vi "GetCCIDInfo.vi"(5 "table name":string="CCID", 6 "Slot":T1, 10 "SerNO":string, 11 "CCID":string) -> (2 "CCID信息":string[](array[string]))   [LabVIEW 2013]
uses:
  SystemCode/SysControl/Slot.ctl
  GlobalValue.vi
panel:
  out "x >= y? 2":bool
  out "子数组":string[](array[string])
  out "x = y?":bool
  out "x >= y?":bool
  out "SerNO OUT":string[](array[string])
  out "CCID 2":string
  out "ID":string
  out "SerNO":string
  out "OUTdata":string[][](array[string])
  out "MainViPath":path
  out "error out":errorcluster caption="错误输出"
  in  "error in (no error)":errorcluster caption="错误输入（无错误）"
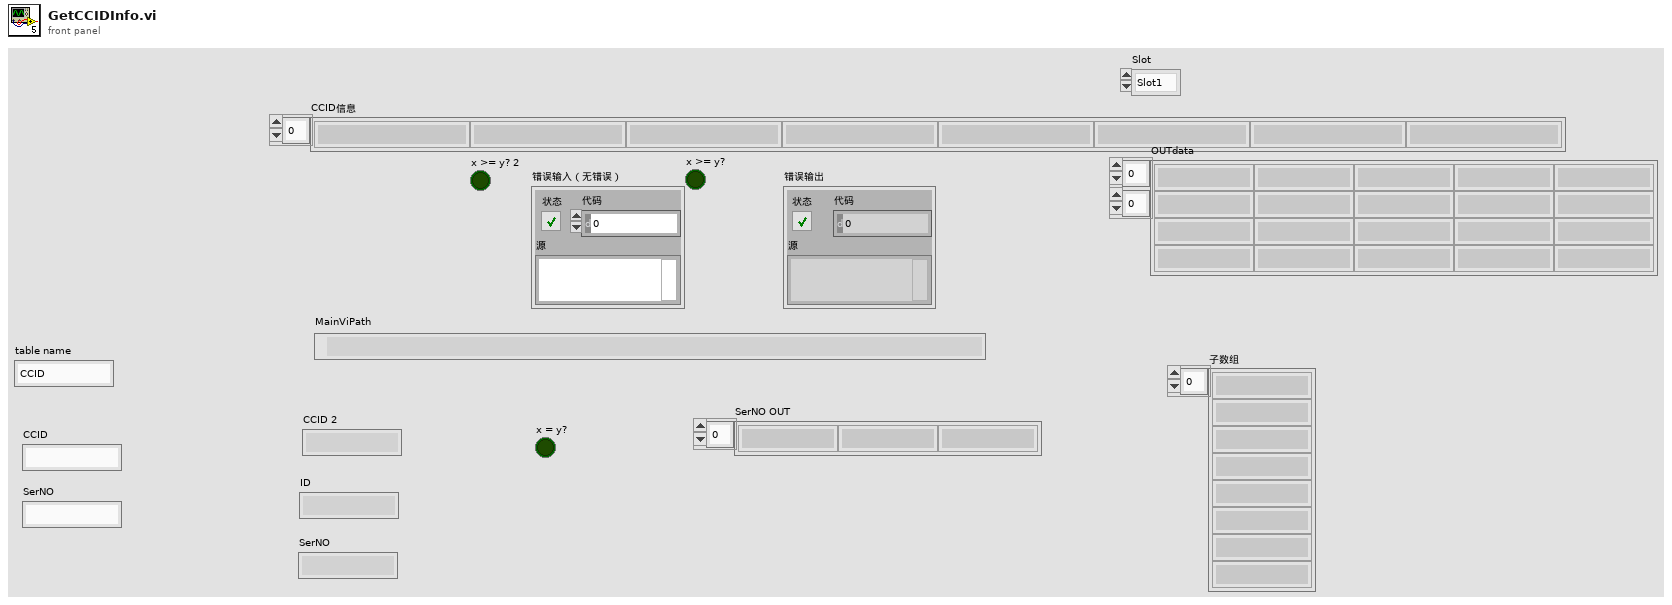
[diagram p1: front panel]
types:
  T1 = typedef "Slot.ctl" = enum16{"Slot1", "Slot2", "Slot3", "Slot4"}
  T2 = enum16{"open", "replace", "create", "open or create", "replace or create", "replace or create with confirmation"}
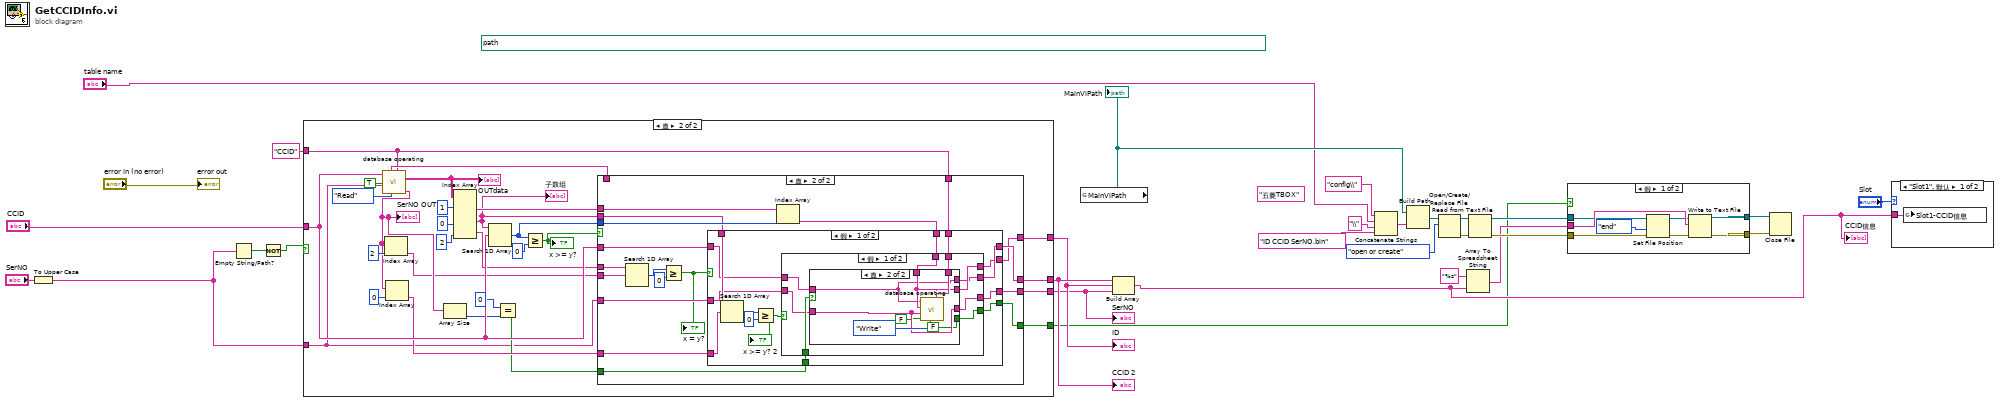
[diagram p0: block diagram]
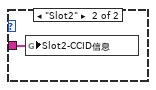
[diagram p3: hidden frame]
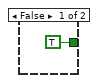
[diagram p4: hidden frame]
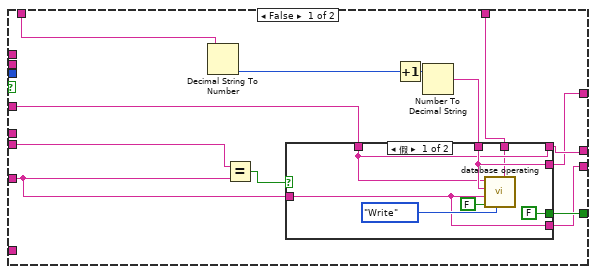
[diagram p5: hidden frame]
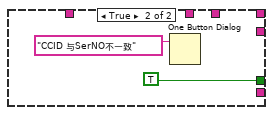
[diagram p6: hidden frame]
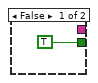
[diagram p7: hidden frame]
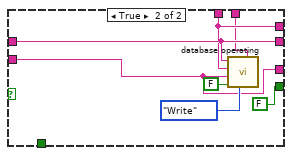
[diagram p8: hidden frame]
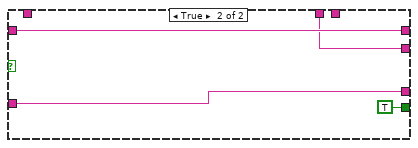
[diagram p9: hidden frame]
diagram:
  (unwired) "五菱TBOX" ("字符串")
  (unwired) path "C:/Documents and Settings/DELL/桌面/homework/五菱T-BOX labview 设计/成品测试/2016-0831 new version/五菱T-BOX TestSystem(增加硬件版本)/五菱T-BOX TestSystem(增加硬件版本)" ("基路径")
  n1 = To Upper Case(1:"SerNO") -> (0:w21:string)
  n2 = Empty String/Path?(string/path=w21) -> (empty?=w23:bool)
  n3 = Not(x=w23) -> (.not. x?=w22:bool)
  n4 = case shown="真" w22 {
    tunnel: "CCID" -> [_ w43]
    tunnel: [_ w57] -> w27
    tunnel: [_ w56] -> w26
    tunnel: [_ w55] -> w25
    tunnel: [TRUE w54] -> w4
    tunnel: w21 -> [_ w32]
    tunnel: "CCID" -> [_ w33]
    frame False {
    }
    frame True {
      n5 = call "database operating.vi"("table name"=w33, "Read or Write"=enum16{"Read", "Write"}."Read", "布尔"=TRUE, "SerNO"=w32, "CCID"=w43) -> ("SerNO OUT"=w38:string[], "OUTdata"=w49:string[][], "OUT MAXID"=w53:string)  [unwired: 4 in]
      "OUTdata" <- w49
      "SerNO OUT" <- w38
      n6 = Index Array(array=w38, index=2 ("索引")) -> (element=w31:string)
      n7 = Index Array(array=w38, index=0 ("索引")) -> (element=w39:string)
      n8 = Array Size(array=w38) -> (size(s)=w37:i32)
      n9 = Index Array(array=w49, index (col) #1=1 ("禁用的索引 (列)"), index (col) #2=0 ("索引 (列)"), index (col) #3=2 ("索引 (列)")) -> (element #1=w48:string[], element #2=w41:string[], element #3=w42:string[])  [unwired: 3 in]
      "子数组" <- w41
      n10 = Search 1D Array(1D array=w41, element=w43) -> (index of element=w50:i32)  [unwired: 1 in]
      n11 = Equal?(x=0, y=w37) -> (x = y?=w35:bool)
      n12 = Greater Or Equal?(x=w50, y=0) -> (x >= y?=w51:bool)
      "x >= y?" <- w51
      n13 = case shown="真" w51 {
        tunnel: w50 -> [_ w92]
        tunnel: w43 -> [w69 w91]
        tunnel: w32 -> [w62 w90]
        tunnel: [w67 w97] -> w57
        tunnel: [w59 w96] -> w56
        tunnel: [w66 w95] -> w55
        tunnel: [w70 w94] -> w54
        tunnel: w53 -> [w65 _]
        tunnel: w48 -> [_ w93]
        tunnel: w42 -> [_ w89]
        tunnel: w31 -> [w63 w84]
        tunnel: w41 -> [_ w85]
        tunnel: w39 -> [_ w83]
        tunnel: w35 -> [_ w82]
        tunnel: w33 -> [w60 w81]
        frame False {
          n14 = Decimal String To Number(string=w65) -> (number=w64:i32)  [unwired: 2 in, 1 out]
          n15 = Equal?(x=w63, y=w62) -> (x = y?=w61:bool)
          n16 = Increment(x=w64) -> (x+1=w71:i32)
          n17 = Number To Decimal String(number=w71) -> (decimal integer string=w68:string)  [unwired: 1 in]
          n18 = case shown="假" w61 {
            tunnel: [FALSE TRUE] -> w70
            tunnel: w69 -> [w75 _]
            tunnel: w68 -> [w77 _]
            tunnel: w62 -> [w74 _]
            tunnel: [w77 _] -> w59
            tunnel: [w75 _] -> w67
            tunnel: [w74 _] -> w66
            tunnel: w60 -> [w72 _]
            frame False {
              n19 = call "database operating.vi"("table name"=w72, "Read or Write"=enum16{"Read", "Write"}."Write", "布尔"=FALSE, "SerNO"=w74, "ID"=w77, "CCID"=w75) -> ()  [unwired: 3 in, 3 out]
            }
            frame True {
              n20 = One Button Dialog(message="CCID 与SerNO不一致" ("消息")) -> ()  [unwired: 1 in, 1 out]
            }
          }
        }
        frame True {
          n21 = Search 1D Array(1D array=w89, element=w84) -> (index of element=w88:i32)  [unwired: 1 in]
          n22 = Greater Or Equal?(x=w88, y=0) -> (x >= y?=w86:bool)
          "x = y?" <- w86
          n23 = Index Array(array=w93, index=w92) -> (element=w98:string)
          n24 = case shown="假" w86 {
            tunnel: w91 -> [w105 w140]
            tunnel: w98 -> [w111 w139]
            tunnel: [w103 w140] -> w97
            tunnel: [w102 w139] -> w96
            tunnel: [w101 w138] -> w95
            tunnel: [w112 TRUE ("布尔")] -> w94
            tunnel: w90 -> [w104 w138]
            tunnel: w85 -> [w109 _]
            tunnel: w83 -> [w110 _]
            tunnel: w82 -> [w100 _]
            tunnel: w81 -> [w99 _]
            frame False {
              n25 = Search 1D Array(1D array=w109, element=w110) -> (index of element=w108:i32)  [unwired: 1 in]
              n26 = Greater Or Equal?(x=w108, y=0) -> (x >= y?=w106:bool)
              "x >= y? 2" <- w106
              n27 = case shown="假" w106 {
                tunnel: [w114 FALSE ("布尔")] -> w112
                tunnel: w111 -> [w118 w133]
                tunnel: w105 -> [w119 w134]
                tunnel: w104 -> [w120 w132]
                tunnel: [w116 w134] -> w103
                tunnel: [w117 w133] -> w102
                tunnel: [w115 w132] -> w101
                tunnel: w100 -> [w121 _]
                tunnel: w99 -> [w113 w130]
                frame False {
                  n28 = case shown="真" w121 {
                    tunnel: w120 -> [_ w128]
                    tunnel: w119 -> [_ w123]
                    tunnel: w118 -> [_ w124]
                    tunnel: [_ w124] -> w117
                    tunnel: [_ w123] -> w116
                    tunnel: [_ w128] -> w115
                    tunnel: [TRUE ("布尔") FALSE ("布尔")] -> w114
                    tunnel: w113 -> [_ w125]
                    frame False {
                    }
                    frame True {
                      n29 = call "database operating.vi"("table name"=w125, "Read or Write"=enum16{"Read", "Write"}."Write", "布尔"=FALSE, "SerNO"=w128, "ID"=w124, "CCID"=w123) -> ()  [unwired: 3 in, 3 out]
                    }
                  }
                }
                frame True {
                  n30 = call "database operating.vi"("table name"=w130, "Read or Write"=enum16{"Read", "Write"}."Write", "布尔"=FALSE, "SerNO"=w132, "ID"=w133, "CCID"=w134) -> ()  [unwired: 3 in, 3 out]
                }
              }
            }
            frame True {
            }
          }
        }
      }
    }
  }
  "SerNO" <- w25
  "ID" <- w26
  "CCID 2" <- w27
  n31 = global read "GlobalValue.vi" "MainViPath"() -> (w3:path)
  "MainViPath" <- w3
  n32 = Build Array(w27, w26, w25) -> (w5:string[])
  "CCID信息" <- w5
  n33 = Concatenate Strings("config\\" ("连接的字符串"), "table name", "\\" ("字符串"), "ID CCID SerNO.bin" ("连接的字符串")) -> (w10:string)
  n34 = Build Path(base path=w3, name or relative path=w10) -> (appended path=w11:path)
  n35 = Open/Create/Replace File(file path (use dialog)=w11, operation (0:open)=T2."open or create" ("操作(0:open)")) -> (refnum out=w14:refnum<file>, error out=w13:errorcluster)  [unwired: 4 in, 1 out]
  n36 = Array To Spreadsheet String(array=w5, 3:"%s" ("格式字符串")) -> (spreadsheet string=w15:string)  [unwired: 1 in]
  n37 = Read from Text File(file (use dialog)=w14, error in=w13) -> (refnum out=w19:refnum<file>, error out=w20:errorcluster)  [unwired: 2 in, 2 out]
  n38 = case shown="假" w4 {
    tunnel: w15 -> [w148 _]
    tunnel: w19 -> [w147 w149]
    tunnel: w20 -> [w143 w150]
    tunnel: [w142 w150] -> w17
    tunnel: [w141 w149] -> w18
    frame False {
      n39 = Set File Position(refnum=w147, from (0:start)=enum16{"start", "end", "current"}."end" ("自（0:起始）"), error in=w143) -> (refnum out=w146:refnum<file>, error out=w145:errorcluster)  [unwired: 1 in]
      n40 = Write to Text File(file (use dialog)=w146, text=w148, error in=w145) -> (refnum out=w141:refnum<file>, error out=w142:errorcluster)  [unwired: 1 in, 1 out]
    }
    frame True {
    }
  }
  n41 = Close File(refnum=w18, error in=w17) -> ()  [unwired: 2 out]
  n42 = case shown="\"Slot1\", 默认" "Slot" {
    tunnel: w5 -> [w151 w152]
    frame "Slot1", Default {
      n43 = global write "GlobalValue.vi" "Slot1-CCID信息"(w151) -> ()
    }
    frame "Slot2" {
      n44 = global write "GlobalValue.vi" "Slot2-CCID信息"(w152) -> ()
    }
  }
  "error out" <- "error in (no error)"
